vi "get_name.vi"(8 "error in (no error)":errorcluster, 11 "ClassB in":refnum<class "ClassB.lvclass">) -> (0 "error out":errorcluster, 2 "name":string="ClassB", 3 "ClassB out":refnum<class "ClassB.lvclass">)   [LabVIEW 2010, in "ClassB.lvclass"]
uses:
  ClassB.lvclass
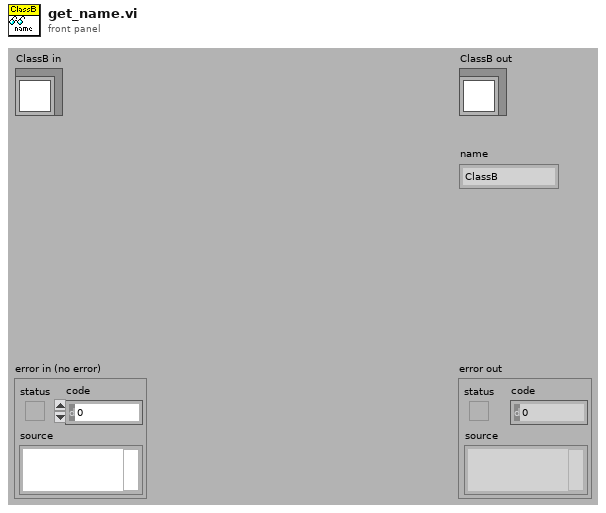
[diagram p1: front panel]
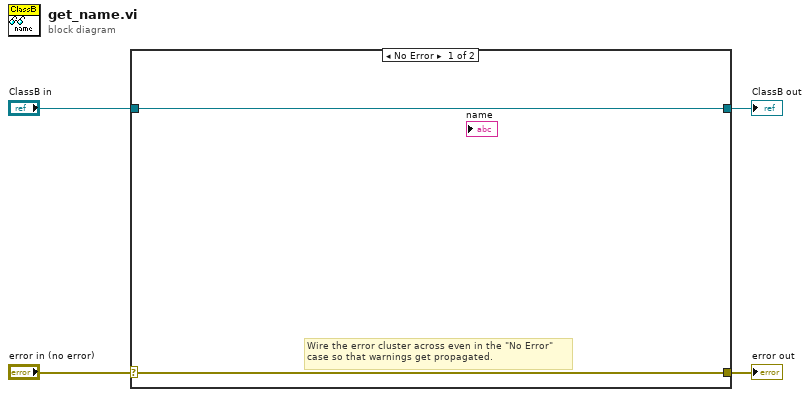
[diagram p0: block diagram]
diagram:
  n1 = case shown="No Error" "error in (no error)" {
    selector: "error in (no error)" -> [w5 w8]
    tunnel: [w5 w8] -> w3
    tunnel: [w6 w7] -> w1
    tunnel: "ClassB in" -> [w6 w7]
    frame No Error {
      # "Wire the error cluster across even in the \"No Error\"\ncase so that warnings get propagated."
    }
    frame Error {
    }
  }
  "error out" <- w3
  "ClassB out" <- w1
